vi "Arm_XBOX.vi"() -> ()   [LabVIEW 2017]
uses:
  <vilib>/MakerHub/Xbox-One-Controller/Public/Open First Controller.vi
  <vilib>/MakerHub/Xbox-One-Controller/LMH-Xbox-One-Controller.lvlib
  <vilib>/LabVIEW Interface for Arduino/LabVIEW Interface for Arduino.lvlib
panel:
  out "Gauge":dbl(knob) scale=0.0..180.0
  out "Shoulder":dbl(knob) scale=-5.0..5.0
  out "Elbow":dbl(knob) scale=-5.0..5.0
  out "BASE VELOCITY CONTROLL":dbl(knob)
  out "Wrist DOWN(A)":bool
  out "Wrist UP(Y)":bool
  out "Grip(VIEW)":bool
  out "Release(MENU)":bool
  out "ELBOW JOINT VELOCITY":dbl(knob) scale=-33000.0..33000.0
  out "SHOULDER JOINT VELOCITY":dbl(knob) scale=-33000.0..33000.0
  in  "STOP":bool
  in  "WRIST PIN":u8=2
  in  "GRIPPER PIN":u8=2
  in  "ELBOW PIN":u8=2
  in  "SHOULDER PIN":u8=2
  in  "BASE PIN":u8=2
  in  "ARD Resource":refnum<visa-resource-name>
  # "Robot Arm Control"
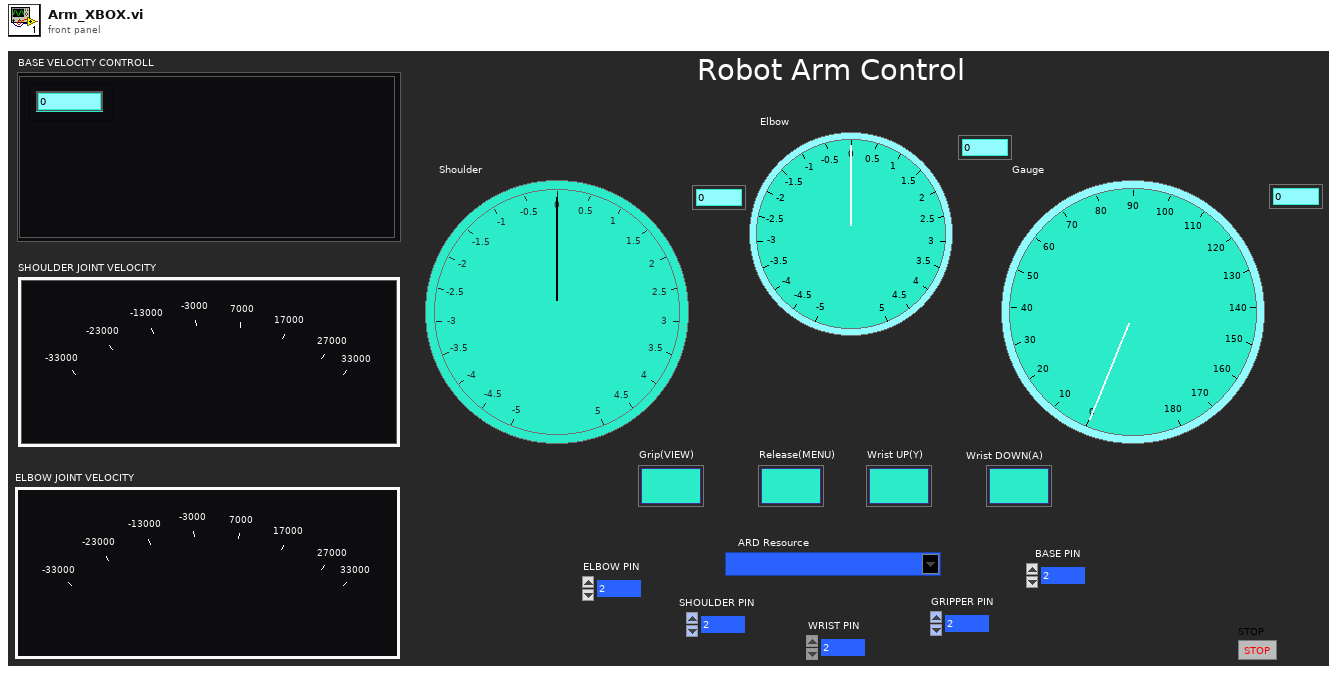
[diagram p1: front panel]
types:
  T1 = typedef "LabVIEW Interface for Arduino.lvlib/Arduino Resource.ctl" = cluster{"VISA resource":refnum<visa-resource-name>, "Board Type":T2, "Connection Type":enum8{"USB / Serial"}, "Bytes Per Packet (15)":u8}
  T2 = typedef "LabVIEW Interface for Arduino.lvlib/Board Type.ctl" = enum16{"Uno", "Dimuelanove w/Atmega 328", "Mega 2560"}
  T3 = typedef "LMH-Xbox-One-Controller.lvlib/Xbox One Controller Ref.ctl" = cluster{"Controller Ref":refnum<k1>, "Event Refnum":refnum<event-registration>, "Worker Ref":refnum<vi>}
  T4 = typedef "LMH-Xbox-One-Controller.lvlib/All Axis Data.ctl" = cluster{"Left Stick":cluster{"X Axis":i32, "Y Axis":i32}, "Right Stick":cluster{"X Axis":i32, "Y Axis":i32}, "Triggers":i32, "D-Pad":T5}
  T5 = typedef "LMH-Xbox-One-Controller.lvlib/DPad Enum.ctl" = enum16{"Idle", "Up", "Up / Right", "Right", "Down / Right", "Down", "Down / Left", "Left", "Up / Left"}
  T6 = typedef "LMH-Xbox-One-Controller.lvlib/All Buttons Visual.ctl" = cluster{"A":T7, "B":T8, "X":T9, "Y":T10, "Left Bumper":T11, "Right Bumper":T12, "View Button":T13, "Menu Button":T14, "Left Stick":T15, "Right Stick":T15}
  T7 = typedef "LMH-Xbox-One-Controller.lvlib/A.ctl" = bool
  T8 = typedef "LMH-Xbox-One-Controller.lvlib/B.ctl" = bool
  T9 = typedef "LMH-Xbox-One-Controller.lvlib/X.ctl" = bool
  T10 = typedef "LMH-Xbox-One-Controller.lvlib/Y.ctl" = bool
  T11 = typedef "LMH-Xbox-One-Controller.lvlib/Left Bumper.ctl" = bool
  T12 = typedef "LMH-Xbox-One-Controller.lvlib/Right Bumper.ctl" = bool
  T13 = typedef "LMH-Xbox-One-Controller.lvlib/View.ctl" = bool
  T14 = typedef "LMH-Xbox-One-Controller.lvlib/Menu.ctl" = bool
  T15 = typedef "LMH-Xbox-One-Controller.lvlib/Thumbstick.ctl" = bool
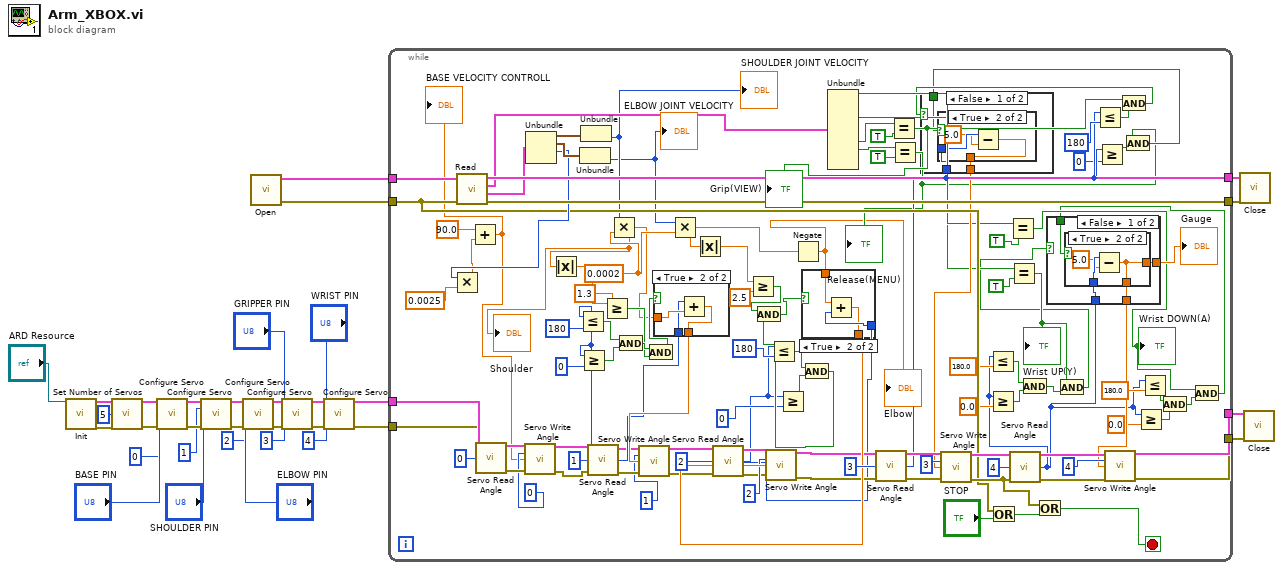
[diagram p0: block diagram]
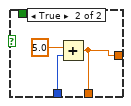
[diagram p3: hidden frame]
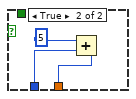
[diagram p5: hidden frame]
diagram:
  n1 = call <vilib>:"Init.vi"("VISA resource"="ARD Resource") -> ("Arduino Resource"=w28:T1, "error out"=w27:errorcluster)  [unwired: 17 in]
  n2 = call <vilib>:"Set Number of Servos.vi"("Arduino Resource"=w28, "Number Of Servos (1)"=u8 5, "error in"=w27) -> ("Arduino Resource"=w26:T1, "error out"=w25:errorcluster)  [unwired: 11 in]
  n3 = call <vilib>:"Configure Servo.vi"("Arduino Resource"=w26, "Servo Number (0)"=u8 0, "DIO Pin (2)"="BASE PIN", "error in"=w25) -> ("Arduino Resource"=w24:T1, "error out"=w23:errorcluster)  [unwired: 10 in]
  n4 = call <vilib>:"Configure Servo.vi"("Arduino Resource"=w24, "Servo Number (0)"=u8 1 ("DIO Pin (2)"), "DIO Pin (2)"="SHOULDER PIN", "error in"=w23) -> ("Arduino Resource"=w22:T1, "error out"=w21:errorcluster)  [unwired: 10 in]
  n5 = call <vilib>:"Configure Servo.vi"("Arduino Resource"=w22, "Servo Number (0)"=u8 2, "DIO Pin (2)"="ELBOW PIN", "error in"=w21) -> ("Arduino Resource"=w20:T1, "error out"=w19:errorcluster)  [unwired: 10 in]
  n6 = call-poly <vilib>:"Open.vi"() -> ("Error Out"=w29:errorcluster, "Xbox One Controller"=w32:T3)  [unwired: 9 in, 1 out]
  n7 = call <vilib>:"Configure Servo.vi"("Arduino Resource"=w20, "Servo Number (0)"=u8 3, "DIO Pin (2)"="GRIPPER PIN", "error in"=w19) -> ("Arduino Resource"=w18:T1, "error out"=w17:errorcluster)  [unwired: 10 in]
  n8 = call <vilib>:"Configure Servo.vi"("Arduino Resource"=w18, "Servo Number (0)"=u8 4, "DIO Pin (2)"="WRIST PIN", "error in"=w17) -> ("Arduino Resource"=w4:T1, "error out"=w3:errorcluster)  [unwired: 10 in]
  n9 = while {
    tunnel: w32 -> [w143]
    tunnel: [w142] -> w31
    tunnel: [w141] -> w30
    tunnel: w29 -> [w84]
    tunnel: w4 -> [w136]
    tunnel: w3 -> [w135]
    tunnel: [w106] -> w2
    tunnel: [w99] -> w1
    stop <- w85 stop-if-true
    w133 = 0.0002
    n10 = call <vilib>:"Read.vi"("Error In"=w84, "Xbox One Controller Ref"=w143) -> ("Error Out"=w141:errorcluster, "All Axis"=w140:T4, "Buttons"=w83:T6, "Xbox One Controller Ref"=w142:T3)  [unwired: 6 in]
    n11 = call <vilib>:"Servo Read Angle.vi"("Arduino Resource"=w136, "Servo Number"=u8 0, "error in"=w135) -> ("Arduino Resource"=w113:T1, "error out"=w105:errorcluster)  [unwired: 10 in, 1 out]
    n12 = Unbundle(w140) -> ("Left Stick"=w139:cluster{"X Axis":i32, "Y Axis":i32}, "Right Stick"=w138:cluster{"X Axis":i32, "Y Axis":i32}, "Triggers"=w123:i32)  [unwired: 1 out]
    n13 = Multiply(x=w123, y=0.0025) -> (x*y=w61:dbl)
    n14 = Add(x=90.0, y=w61) -> (x+y=w56:dbl)
    "BASE VELOCITY CONTROLL" <- w56
    n15 = call <vilib>:"Servo Write Angle.vi"("Arduino Resource"=w113, "Servo Number"=u8 0, "Angle (Degrees)"=w56, "error in"=w105) -> ("Arduino Resource"=w112:T1, "error out"=w104:errorcluster)  [unwired: 10 in]
    n16 = Unbundle(w138) -> ("Y Axis"=w64:i32)  [unwired: 1 out]
    "ELBOW JOINT VELOCITY" <- w64
    n17 = Unbundle(w139) -> ("Y Axis"=w65:i32)  [unwired: 1 out]
    "SHOULDER JOINT VELOCITY" <- w65
    n18 = call <vilib>:"Servo Read Angle.vi"("Arduino Resource"=w112, "Servo Number"=u8 1, "error in"=w104) -> ("Arduino Resource"=w111:T1, "Angle (Degrees)"=w121:u8, "error out"=w103:errorcluster)  [unwired: 10 in]
    n19 = Less Or Equal?(x=w121, y=180) -> (x <= y?=w126:bool)
    n20 = Greater Or Equal?(x=w121, y=0) -> (x >= y?=w127:bool)
    n21 = Multiply(x=w65, y=w133) -> (x*y=w33:dbl)
    "Shoulder" <- w33
    n22 = Absolute Value(x=w33) -> (abs(x)=w58:dbl)
    n23 = Greater Or Equal?(x=w58, y=1.3) -> (x >= y?=w118:bool)
    n24 = And(x=w126, y=w127) -> (x .and. y?=w120:bool)
    n25 = And(x=w120, y=w118) -> (x .and. y?=w119:bool)
    n26 = case shown="True" w119 {
      tunnel: w33 -> [_ w172]
      tunnel: [w169 w170] -> w122
      tunnel: w121 -> [w169 w171]
      frame False {
      }
      frame True {
        n27 = Add(x=w171, y=w172) -> (x+y=w170:dbl)
      }
    }
    n28 = call <vilib>:"Servo Write Angle.vi"("Arduino Resource"=w111, "Servo Number"=u8 1, "Angle (Degrees)"=w122, "error in"=w103) -> ("Arduino Resource"=w110:T1, "error out"=w102:errorcluster)  [unwired: 10 in]
    n29 = Multiply(x=w64, y=w133) -> (x*y=w35:dbl)
    n30 = Absolute Value(x=w35) -> (abs(x)=w57:dbl)
    n31 = call <vilib>:"Servo Read Angle.vi"("Arduino Resource"=w110, "Servo Number"=u8 2, "error in"=w102) -> ("Arduino Resource"=w98:T1, "Angle (Degrees)"=w52:u8, "error out"=w92:errorcluster)  [unwired: 10 in]
    n32 = Greater Or Equal?(x=w57, y=2.5) -> (x >= y?=w116:bool)
    n33 = Less Or Equal?(x=w52, y=180) -> (x <= y?=w124:bool)
    n34 = Greater Or Equal?(x=w52, y=0) -> (x >= y?=w125:bool)
    n35 = Negate(x=w35) -> (-x=w34:dbl)
    "Elbow" <- w34
    n36 = And(x=w124, y=w125) -> (x .and. y?=w117:bool)
    n37 = And(x=w116, y=w117) -> (x .and. y?=w115:bool)
    n38 = case shown="True" w115 {
      tunnel: w34 -> [_ w168]
      tunnel: w52 -> [w165 w167]
      tunnel: [w165 w166] -> w114
      frame False {
      }
      frame True {
        n39 = Add(x=w168, y=w167) -> (x+y=w166:dbl)
      }
    }
    n40 = call <vilib>:"Servo Write Angle.vi"("Arduino Resource"=w98, "Servo Number"=u8 2, "Angle (Degrees)"=w114, "error in"=w92) -> ("Arduino Resource"=w97:T1, "error out"=w96:errorcluster)  [unwired: 10 in]
    n41 = Unbundle(w83) -> ("A"=w77:T7, "Y"=w76:T10, "View Button"=w82:T13, "Menu Button"=w81:T14)  [unwired: 6 out]
    n42 = call <vilib>:"Servo Read Angle.vi"("Arduino Resource"=w97, "Servo Number"=u8 3, "error in"=w96) -> ("Arduino Resource"=w109:T1, "Angle (Degrees)"=w69:u8, "error out"=w101:errorcluster)  [unwired: 10 in]
    n43 = Equal?(x=w82, y=TRUE) -> (x = y?=w63:T13)
    "Grip(VIEW)" <- w63
    n44 = Equal?(x=w81, y=TRUE) -> (x = y?=w62:T14)
    "Release(MENU)" <- w62
    n45 = Or(x=w84, y="STOP") -> (x .or. y?=w87:bool)
    n46 = Equal?(x=w77, y=TRUE) -> (x = y?=w37:T7)
    "Wrist DOWN(A)" <- w37
    n47 = Equal?(x=w76, y=TRUE) -> (x = y?=w46:T10)
    "Wrist UP(Y)" <- w46
    n48 = Less Or Equal?(x=w69, y=u8 180) -> (x <= y?=w71:bool)
    n49 = Greater Or Equal?(x=w69, y=u8 0) -> (x >= y?=w67:bool)
    n50 = And(x=w63, y=w71) -> (x .and. y?=w70:T13)
    n51 = And(x=w62, y=w67) -> (x .and. y?=w66:T14)
    n52 = case shown="False" w70 {
      tunnel: w69 -> [w157 w164]
      tunnel: [w156 w162] -> w78
      tunnel: w66 -> [w155 _]
      frame False {
        n53 = case shown="True" w155 {
          tunnel: w157 -> [w158 w160]
          tunnel: [w158 w161] -> w156
          frame False {
          }
          frame True {
            n54 = Subtract(x=w160, y=5.0 ("x")) -> (x-y=w161:dbl)
          }
        }
      }
      frame True {
        n55 = Add(x=u8 5, y=w164) -> (x+y=w162:u8)
      }
    }
    n56 = call <vilib>:"Servo Write Angle.vi"("Arduino Resource"=w109, "Servo Number"=u8 3, "Angle (Degrees)"=w78, "error in"=w101) -> ("Arduino Resource"=w108:T1, "error out"=w86:errorcluster)  [unwired: 10 in]
    n57 = call <vilib>:"Servo Read Angle.vi"("Arduino Resource"=w108, "Servo Number"=u8 4, "error in"=w86) -> ("Arduino Resource"=w107:T1, "Angle (Degrees)"=w41:u8, "error out"=w100:errorcluster)  [unwired: 10 in]
    n58 = Less Or Equal?(x=w41, y=180.0) -> (x <= y?=w49:bool)
    n59 = Greater Or Equal?(x=w41, y=0.0) -> (x >= y?=w48:bool)
    n60 = And(x=w49, y=w48) -> (x .and. y?=w47:bool)
    n61 = Or(x=w86, y=w87) -> (x .or. y?=w85:bool)
    n62 = And(x=w46, y=w47) -> (x .and. y?=w45:T10)
    n63 = Greater Or Equal?(x=w41, y=0.0) -> (x >= y?=w40:bool)
    n64 = Less Or Equal?(x=w41, y=180.0) -> (x <= y?=w39:bool)
    n65 = And(x=w39, y=w40) -> (x .and. y?=w38:bool)
    n66 = And(x=w37, y=w38) -> (x .and. y?=w36:T7)
    n67 = case shown="False" w45 {
      tunnel: w41 -> [w147 w154]
      tunnel: [w146 w153] -> w73
      tunnel: [w145 w153] -> w44
      tunnel: w36 -> [w144 _]
      frame False {
        n68 = case shown="True" w144 {
          tunnel: w147 -> [w148 w150]
          tunnel: [w148 w151] -> w146
          tunnel: [w148 w151] -> w145
          frame False {
          }
          frame True {
            n69 = Subtract(x=w150, y=5.0 ("x")) -> (x-y=w151:dbl)
          }
        }
      }
      frame True {
        n70 = Add(x=5.0, y=w154) -> (x+y=w153:dbl)
      }
    }
    "Gauge" <- w44
    n71 = call <vilib>:"Servo Write Angle.vi"("Arduino Resource"=w107, "Servo Number"=u8 4, "Angle (Degrees)"=w73, "error in"=w100) -> ("Arduino Resource"=w106:T1, "error out"=w99:errorcluster)  [unwired: 10 in]
  }
  n72 = call <vilib>:"Close.vi"("Error In"=w30, "Xbox One Controller Ref"=w31) -> ()  [unwired: 9 in, 1 out]
  n73 = call <vilib>:"Close.vi"("Arduino Resource"=w2, "error in"=w1) -> ()  [unwired: 13 in, 1 out]
